vi "GitDiffNowWithMaster.vi"(8 "error in (no error)":errorcluster, 9 "Save Repo Path":path=path "", 10 "Save Cluster":T1 {"Select Layout" items=["Default"]}, 11 "Git exec":string="git") -> (0 "error out":errorcluster, 1 "Save Repo Path Out":path, 2 "Save Cluster Out":T1 {"Select Layout" items=["Default"]}, 3 "Git exec out":string="git", 4 "Diff Output":string, 5 "Differ":bool)   [LabVIEW 2013]
uses:
  TypeDefs/SaveCluster.ctl
  VariableManagerCodes/VariableManager/VariableManager.lvclass
  DeviceVIs/Device/Device.lvclass
  <vilib>/Utility/miscctls.llb/LVStringsAndValuesArrayTypeDef_I32.ctl
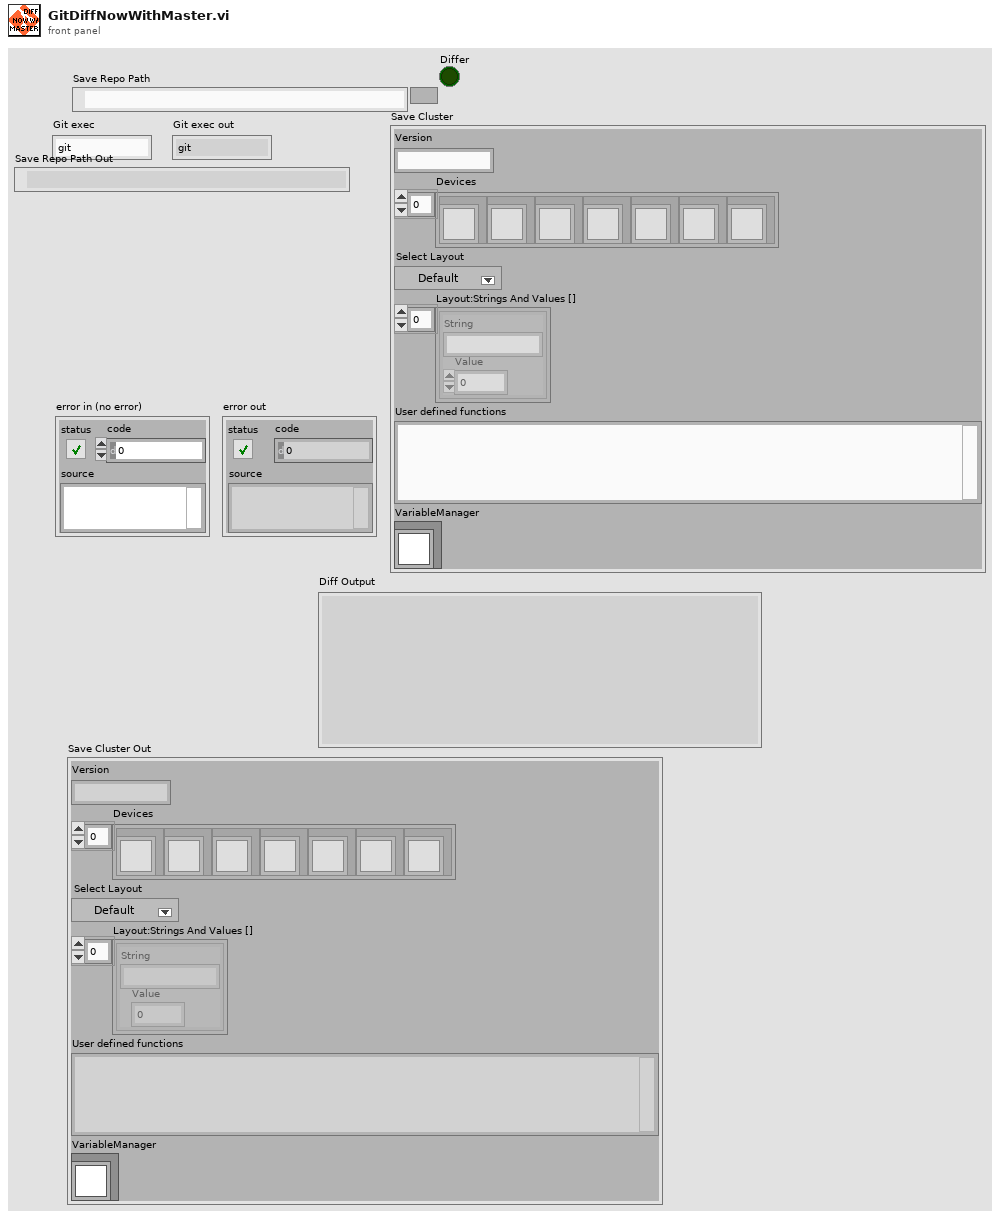
[diagram p1: front panel]
types:
  T1 = typedef "SaveCluster.ctl" = cluster{"Version":string, "Devices":refnum<class "Device.lvclass">[], "Select Layout":i32, "Layout:Strings And Values []":T2, "User defined functions":string, "VariableManager":refnum<class "VariableManager.lvclass">}
  T2 = typedef "LVStringsAndValuesArrayTypeDef_I32.ctl" = cluster{"String":string, "Value":i32}[]
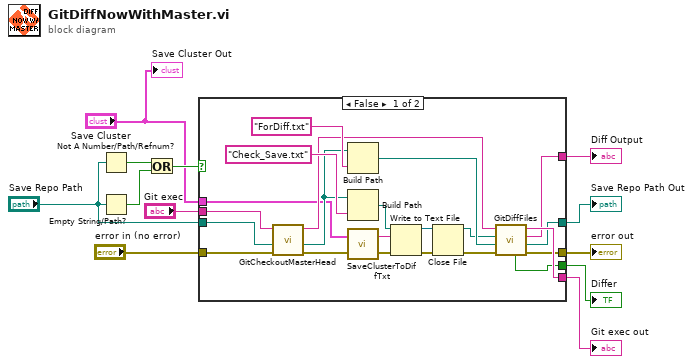
[diagram p0: block diagram]
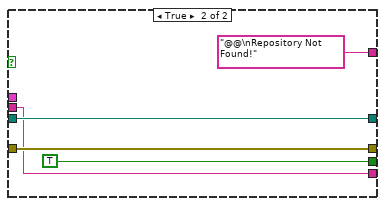
[diagram p2: hidden frame]
diagram:
  n1 = Not A Number/Path/Refnum?(number/path/refnum="Save Repo Path") -> (NaN/Path/Refnum?=w10:bool)
  n2 = Empty String/Path?(string/path="Save Repo Path") -> (empty?=w9:bool)
  n3 = Or(x=w10, y=w9) -> (x .or. y?=w8:bool)
  n4 = case shown="False" w8 {
    tunnel: "error in (no error)" -> [w19 w38]
    tunnel: [w24 w38] -> w5
    tunnel: "Save Repo Path" -> [w15 w37]
    tunnel: [w23 w37] -> w4
    tunnel: "Git exec" -> [w16 w35]
    tunnel: [w27 w35] -> w6
    tunnel: [w22 "@@\nRepository Not Found!" ("Response")] -> w3
    tunnel: [w21 TRUE ("Differ")] -> w2
    tunnel: "Save Cluster" -> [w13 _]
    frame False {
      n5 = call "GitCheckoutMasterHead.vi"("error in (no error)"=w19, "File"=w15, "Git exec"=w16) -> ("error out"=w18:errorcluster, "File out"=w14:path, "Git exec out"=w17:string)  [unwired: 5 in, 1 out]
      n6 = Build Path(base path=w14, name or relative path="ForDiff.txt") -> (appended path=w26:path)
      n7 = Build Path(base path=w14, name or relative path="Check_Save.txt") -> (appended path=w32:path)
      n8 = call "SaveClusterToDiffTxt.vi"("Save Cluster"=w13) -> ("DiffText"=w30:string)  [unwired: 2 in]
      n9 = Write to Text File(file (use dialog)=w32, text=w30, error in=w18) -> (refnum out=w31:refnum<file>, error out=w29:errorcluster)  [unwired: 1 in, 1 out]
      n10 = Close File(refnum=w31, error in=w29) -> (path=w25:path, error out=w28:errorcluster)
      n11 = call "GitDiffFiles.vi"("error in (no error)"=w28, "Old File"=w26, "New File"=w25, "Git exec"=w17) -> ("error out"=w24:errorcluster, "Old File out"=w23:path, "Response"=w22:string, "Git exec out"=w27:string, "Differ"=w21:bool)  [unwired: 3 in]
    }
    frame True {
    }
  }
  "Git exec out" <- w6
  "error out" <- w5
  "Diff Output" <- w3
  "Save Repo Path Out" <- w4
  "Differ" <- w2
  "Save Cluster Out" <- "Save Cluster"
